vi "Set input current_ChAmmeter.vi"(0 "the lower limit for the voltage":dbl=1.0, 1 "accuracy (input)":dbl step=0.01, 4 "4070_address":refnum<k15>="PXI3Slot5_5 (8)" caption="4070_out", 5 "Start voltage":dbl=3.0 format="%#.7f", 9 "the upper limit for the voltage":dbl=5.0, 11 "instrument handle":refnum<k15>, 12 "the optimum current(input)":dbl format="%#_6f", 14 "res(input)":dbl=110.0, 15 "channel name":string) -> (3 "accommodated voltage (out)":dbl, 6 "Error message":string, 10 "current value, mA":dbl, 13 "the voltage drop across the resistor":dbl=1.1)   [LabVIEW 2013]
uses:
  <instrlib>/niDMM/nidmm.llb/niDMM Resolution in Digits.ctl
  <instrlib>/niDMM/nidmm.llb/niDMM Function.ctl
  <vilib>/Analysis/baseanly.llb/Mean (DBL).vi
  <instrlib>/niDMM/nidmm.llb/niDMM Configure Measurement Digits.vi
  <vilib>/Analysis/NI_AALBase.lvlib
panel:
  out "CH1_Uпит, mA":dbl=15.418111291908591 caption="CH1_AO, ìA" format="%_6g"
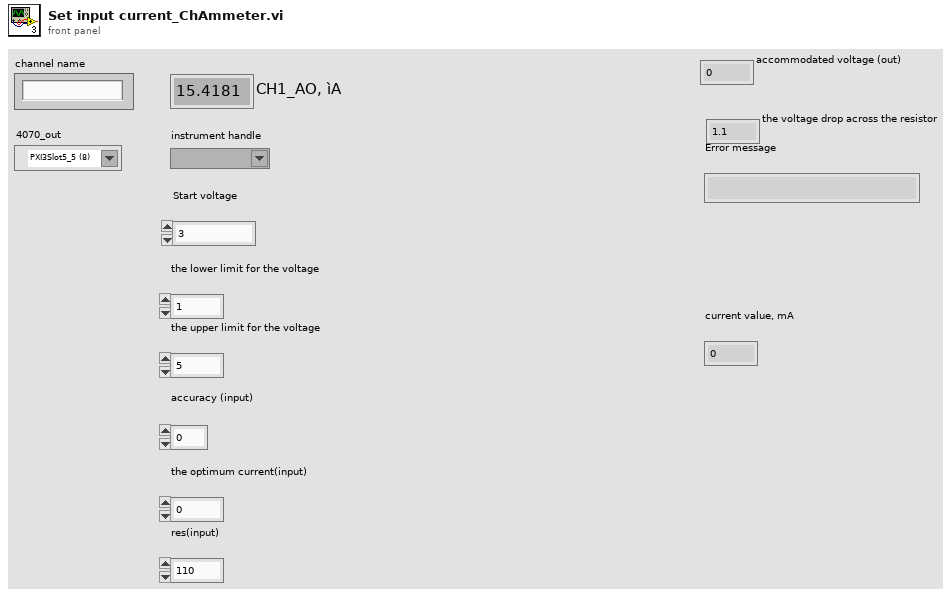
[diagram p1: front panel]
types:
  T1 = typedef "niDMM Function.ctl" = enum16{"DC Volts", "AC Volts", "DC Current", "AC Current", "2-wire Resistance", "4-wire Resistance", "Diode", "Frequency", "Period", "AC Volts DC Coupled", "Capacitance", "Inductance", "Temperature"}
  T2 = typedef "niDMM Resolution in Digits.ctl" = dbl
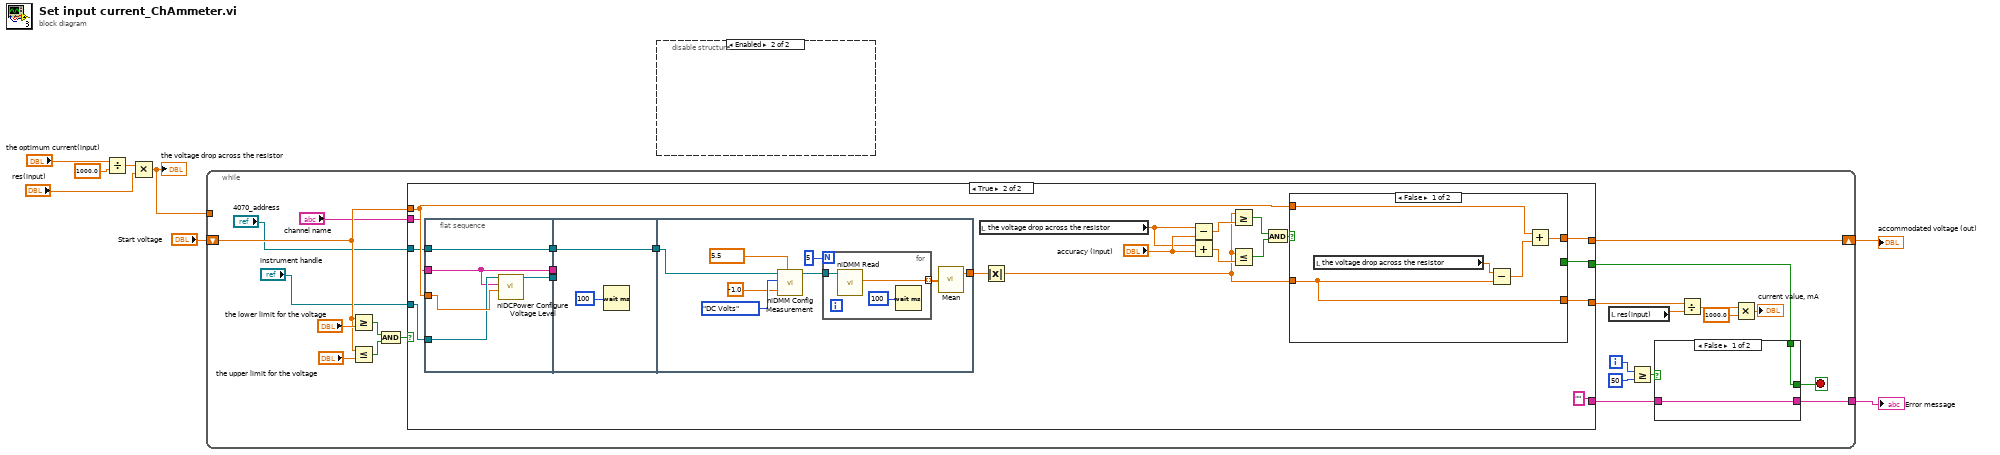
[diagram p0: block diagram]
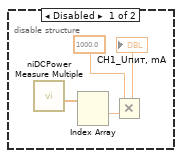
[diagram p2: hidden frame]
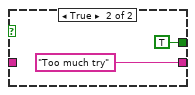
[diagram p3: hidden frame]
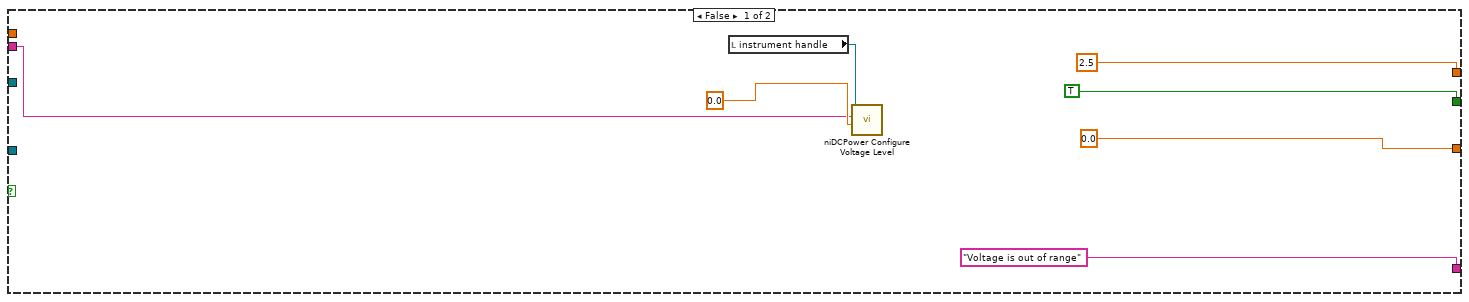
[diagram p4: hidden frame]
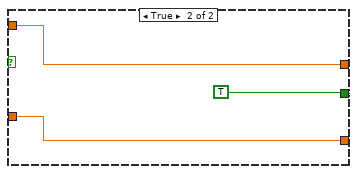
[diagram p5: hidden frame]
diagram:
  n1 = Divide(x="the optimum current(input)", y=1000.0) -> (x/y=w5:dbl)
  n2 = Multiply(x=w5, y="res(input)") -> (x*y=w1:dbl)
  "the voltage drop across the resistor" <- w1
  n3 = while {
    tunnel: [w14] -> w8
    shift-right: [w20] -> w2
    shift-left: "Start voltage" -> [w21]
    tunnel: w1 -> [_]
    i -> [w17]
    stop <- w13 stop-if-true
    n4 = Greater Or Equal?(x=w21, y="the lower limit for the voltage") -> (x >= y?=w29:bool)
    n5 = Less Or Equal?(x=w21, y="the upper limit for the voltage") -> (x <= y?=w30:bool)
    n6 = And(x=w29, y=w30) -> (x .and. y?=w26:bool)
    n7 = case shown="True" w26 {
      tunnel: ["Voltage is out of range" ""] -> w15
      tunnel: [2.5 ("accommodated voltage") w54] -> w20
      tunnel: [TRUE w60] -> w12
      tunnel: [0.0 w55] -> w19
      tunnel: w21 -> [_ w50]
      tunnel: "instrument handle" -> [_ w48]
      tunnel: "channel name" -> [w35 w47]
      tunnel: "4070_address" -> [_ w45]
      frame False {
        n8 = local read "instrument handle"() -> (w37:refnum<k15>)
        n9 = call <instrlib>:"niDCPower Configure Voltage Level.vi"("voltage level"=0.0, "channel name"=w35, "instrument handle"=w37) -> ()  [unwired: 7 in, 2 out]
      }
      frame True {
        n10 = flat-sequence {
          tunnel: w50 -> [w66]
          tunnel: [w67] -> w51
          tunnel: [w64] -> w49
          tunnel: w48 -> [w65]
          tunnel: w47 -> [w64]
          tunnel: [w63] -> w46
          tunnel: w45 -> [w63]
          tunnel: w51 -> [_]
          tunnel: w49 -> [_]
          tunnel: w46 -> [w68]
          tunnel: [w68] -> w44
          tunnel: w44 -> [w71]
          tunnel: [w70] -> w43
          frame #0 {
            n11 = call <instrlib>:"niDCPower Configure Voltage Level.vi"("voltage level"=w66, "channel name"=w64, "instrument handle"=w65) -> ("instrument handle out"=w67:refnum<k15>)  [unwired: 7 in, 1 out]
          }
          frame #1 {
            n12 = Wait (ms)(milliseconds to wait=u32 100) -> ()  [unwired: 1 out]
          }
          frame #2 {
            w74 = T2 5.5 items=["3 1/2"=3.5, "4 1/2"=4.5, "5 1/2"=5.5, "6 1/2"=6.5, "7 1/2"=7.5] ("Resolution in Digits")
            n13 = call-poly <instrlib>:"niDMM Config Measurement.vi"("Range"=-1.0 ("Configuration:Measurement Options:Max Frequency"), "Resolution in Digits"=w74, "Function"=niDMM_Function."DC Volts" ("multimeter mode"), "instrument handle"=w71) -> ("instrument handle out"=w75:refnum<k15>)  [unwired: 6 in, 1 out]
            n14 = for {
              N: 5 -> [_]
              tunnel: w75 -> [w79]
              tunnel: [w78] -> w76 mode=indexing
              n15 = call <instrlib>:"niDMM Read.vi"("instrument handle"=w79) -> ("Measurement"=w78:dbl)  [unwired: 8 in, 2 out]
              n16 = Wait (ms)(milliseconds to wait=u32 100) -> ()  [unwired: 1 out]
            }
            n17 = call-poly <vilib>:"Mean.vi"("X"=w76) -> ("mean"=w70:dbl)  [unwired: 1 out]
          }
        }
        n18 = local read "the voltage drop across the resistor"() -> (w58:dbl)
        n19 = Absolute Value(x=w43) -> (abs(x)=w42:dbl)
        n20 = Subtract(x=w58, y="accuracy (input)") -> (x-y=w62:dbl)
        n21 = Add(x=w58, y="accuracy (input)") -> (x+y=w61:dbl)
        n22 = Greater Or Equal?(x=w42, y=w62) -> (x >= y?=w56:bool)
        n23 = Less Or Equal?(x=w42, y=w61) -> (x <= y?=w57:bool)
        n24 = And(x=w56, y=w57) -> (x .and. y?=w53:bool)
        n25 = case shown="False" w53 {
          tunnel: [_ TRUE] -> w60
          tunnel: [w84 w86] -> w54
          tunnel: w42 -> [w82 w87]
          tunnel: [w82 w87] -> w55
          tunnel: w50 -> [w83 w86]
          frame False {
            n26 = local read "the voltage drop across the resistor"() -> (w81:dbl)
            n27 = Subtract(x=w81, y=w82) -> (x-y=w85:dbl)
            n28 = Add(x=w83, y=w85) -> (x+y=w84:dbl)
          }
          frame True {
          }
        }
      }
    }
    n29 = local read "res(input)"() -> (w25:dbl)
    n30 = Greater Or Equal?(x=w17, y=50) -> (x >= y?=w18:bool)
    n31 = case shown="False" w18 {
      tunnel: w15 -> [w32 _]
      tunnel: [w32 "Too much try"] -> w14
      tunnel: [w31 TRUE] -> w13
      tunnel: w12 -> [w31 _]
      frame False {
      }
      frame True {
      }
    }
    n32 = Divide(x=w19, y=w25) -> (x/y=w24:dbl)
    n33 = Multiply(x=w24, y=1000.0) -> (x*y=→"current value, mA":dbl)
  }
  "Error message" <- w8
  "accommodated voltage (out)" <- w2
  n34 = disable-structure shown="Enabled" {
    frame Disabled {
      n35 = call <instrlib>:"niDCPower Measure Multiple.vi"() -> ("current measurements"=w89:dbl[])  [unwired: 8 in, 3 out]
      n36 = Index Array(array=w89) -> (element #1=w91:dbl)  [unwired: 2 in, 1 out]
      n37 = Multiply(x=1000.0 ("y"), y=w91) -> (x*y=→"CH1_Uпит, mA":dbl)
    }
    frame Enabled {
    }
  }
